vi "CTRE_Phoenix_CANcoder_ConfigVelocityMeasurementPeriod.vi"(6 "timeoutMs":i32, 8 "error in":errorcluster, 10 "Period":T1=100 items=["Period_1ms"=1, "Period_2ms"=2, "Period_5ms"=5, "Period_10ms"=10, "Period_20ms"=20, "Period_25ms"=25, "Period_50ms"=50, "Period_100ms"=100], 11 "CTRE_CANcoder_DeviceRef":T2) -> (0 "error out":errorcluster, 3 "CTRE_CANcoder_DeviceRef":T2)   [LabVIEW 2020]
doc: "Configures the period of each velocity sample.\nEvery 1ms a position value is sampled, and the delta between that sample and the position sampled kPeriod ms ago is inserted into a filter. kPeriod is configured with this function."
uses:
  <vilib>/Rock Robotics/WPI/ThirdParty/Phoenix-LabVIEW/CANCoder/Controls/CTRE_Phoenix_CANcoder_DeviceRef.ctl
  <vilib>/Rock Robotics/WPI/ThirdParty/Phoenix-LabVIEW/Motor Controller/Controls/CTRE_Phoenix_MotorControl_VelocityMeasurementPeriod.ctl
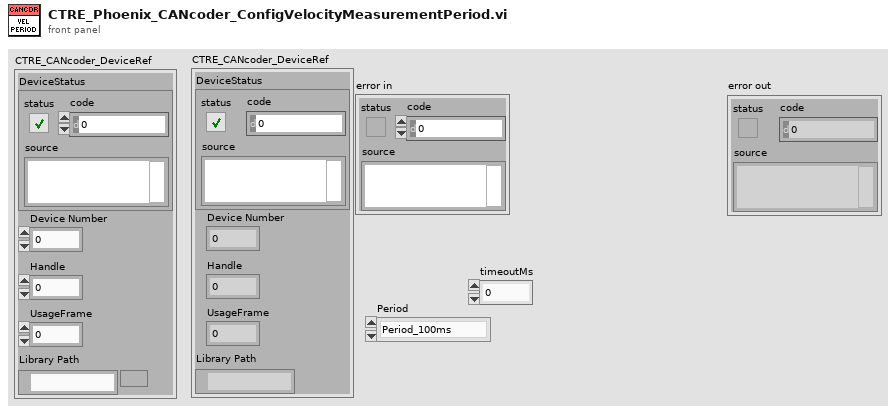
[diagram p1: front panel]
types:
  T1 = typedef "CTRE_Phoenix_MotorControl_VelocityMeasurementPeriod.ctl" = u16
  T2 = typedef "CTRE_Phoenix_CANcoder_DeviceRef.ctl" = cluster{"DeviceStatus":errorcluster, "Device Number":u8, "Handle":u64, "UsageFrame":u32, "Library Path":path}
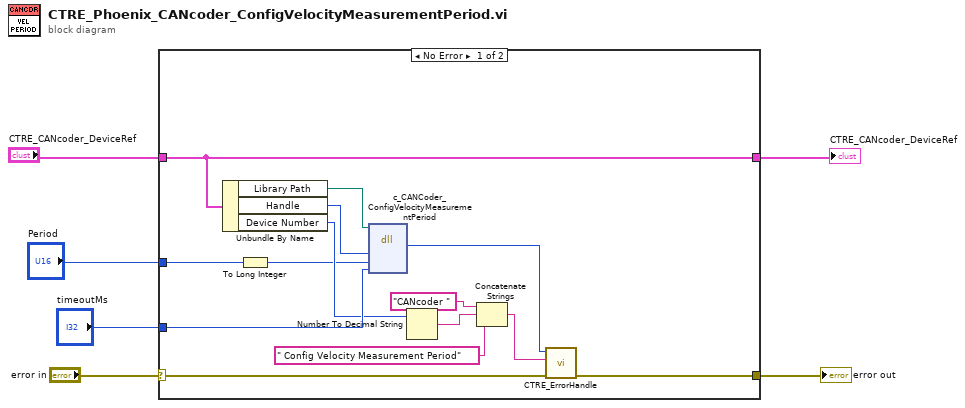
[diagram p0: block diagram]
diagram:
  n1 = case shown="No Error" "error in" {
    selector: "error in" -> [w17 w22]
    tunnel: "CTRE_CANcoder_DeviceRef" -> [w18 w21]
    tunnel: [w16 w22] -> w5
    tunnel: [w18 w21] -> w2
    tunnel: "Period" -> [w14 _]
    tunnel: "timeoutMs" -> [w13 _]
    frame No Error {
      n2 = Unbundle By Name(w18) -> ("Library Path"=w20:path, "Handle"=w19:u64, "Device Number"=w9:u8)
      n3 = To Long Integer(number=w14) -> (32bit integer=w7:i32)
      n4 = dll-call lib="?" fn="c_CANCoder_ConfigVelocityMeasurementPeriod"(path in=w20, "handle"=w19, "period"=w7, "timeoutMs"=w13) -> ("CTR_Code"=w15:i8)  [unwired: 5 in, 2 out]
      n5 = Number To Decimal String(number=w9) -> (decimal integer string=w12:string)  [unwired: 1 in]
      n6 = Concatenate Strings("CANcoder " ("string"), w12, " Config Velocity Measurement Period" ("string")) -> (w10:string)
      n7 = call <vilib>:"CTRE_ErrorHandle.vi"("error in"=w17, "origin"=w10, "code"=w15) -> ("error out"=w16:errorcluster)  [unwired: 8 in]
    }
    frame Error {
    }
  }
  "error out" <- w5
  "CTRE_CANcoder_DeviceRef" <- w2
